vi "Has.vi"(7 "path override":path, 8 "error in (no error)":errorcluster, 11 "capability_":string) -> (0 "error out":errorcluster, 3 "Has":bool)   [LabVIEW 2025, in "libzmq-v143-mt-4_3_6.lvlib"]
doc: "ZMQ_EXPORT int zmq_has (const char *capability_);"
uses:
  libzmq-v143-mt-4_3_6.lvlib
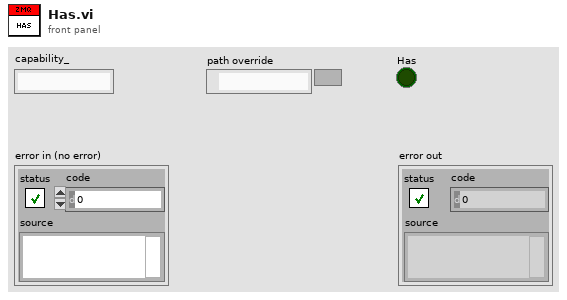
[diagram p1: front panel]
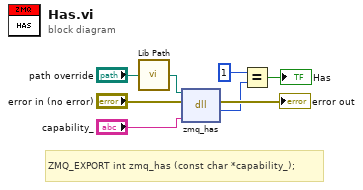
[diagram p0: block diagram]
diagram:
  # "ZMQ_EXPORT int zmq_has (const char *capability_);"
  n1 = call "Lib Path.vi"("path override"="path override") -> ("lib path"=w5:path)
  n2 = dll-call lib="home/james/Documents/ZeroMQ_LV/libzmq-v143-mt-4_3_6/libzmq.so" fn="zmq_has"(path in=w5, error in="error in (no error)", "capability_"="capability_") -> (error out=→"error out":errorcluster, "return type"=w3:i32)  [unwired: 2 in, 1 out]
  n3 = Equal?(x=1, y=w3) -> (x = y?=→"Has":bool)
